vi "Set Actor Error.vi"(5 "Message Postfix":string, 7 "Error Name":T1, 8 "error in (no error)":errorcluster, 11 "Actor in":refnum<class "Ancestral Actor.lvclass">) -> (0 "error out":errorcluster, 3 "Actor out":refnum<class "Ancestral Actor.lvclass">)   [LabVIEW 2016, in "Stream Actor.lvlib" / "Ancestral Actor.lvclass"]
doc: "--\nCopyright © 2017 Composed SystemsI All rights reserved.\n\nAuthor: Jon McBee <jon.mcbee@composed.io>\n\nThis library is provided \"AS IS\" ,WITHOUT WARRANTIES OR\nCONDITIONS OF ANY KIND, either express or implied.\n\nComposed Systems -- composed.io\n\nStream 0.0.1.1\nJon McBee - Composed Systems\nCopyright (c) 2017, Composed Systems"
uses:
  <userlib>/Composed Systems/Stream/Actor/Actor Class/Ancestral Actor.lvclass
  <userlib>/Composed Systems/Stream/Actor/Actor Class/Error Name.ctl
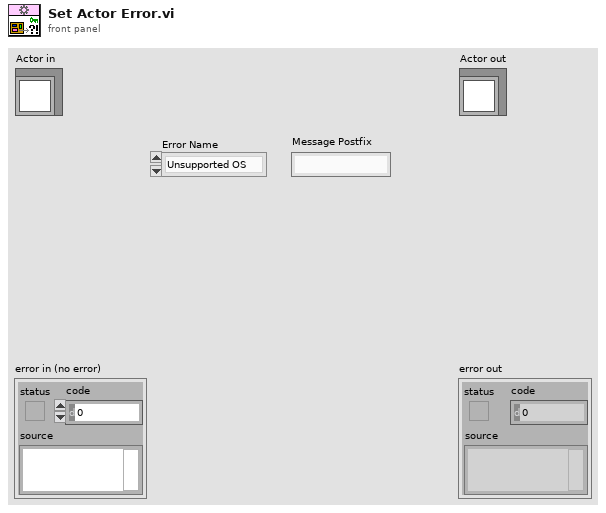
[diagram p1: front panel]
types:
  T1 = typedef "Stream Actor.lvlib/Ancestral Actor.lvclass/Error Name.ctl" = enum16{"Unsupported OS", "Object Already Initialized", "Object Not Initialized", "Method Not Implemented"}
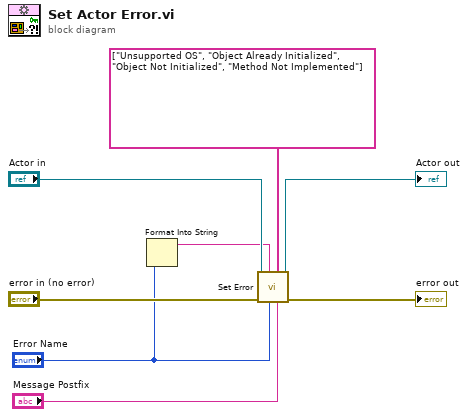
[diagram p0: block diagram]
diagram:
  n1 = Format Into String("Error Name") -> (resulting string=w2:string)  [unwired: 3 in, 1 out]
  n2 = call <userlib>:"Set Error.vi"("Message Postfix"="Message Postfix", "Error Messages"=string[] ["Unsupported OS", "Object Already Initialized", "Object Not Initialized", "Method Not Implemented"], "Error Code"="Error Name", "Error Name"=w2, "error in (no error)"="error in (no error)", "Actor in"="Actor in") -> ("error out"=→"error out":errorcluster, "Actor out"=→"Actor out":refnum<class "Ancestral Actor.lvclass">)  [unwired: 4 in]
